vi "QCA INIT.vi"   [LabVIEW 2019]
doc: "INIT all sections of the QCA. This causes all config files to be reread and all configuration globals written to as if from power up."
uses:
  TPS Global.vi
  QCA Global.vi
  <vilib>/Utility/config.llb/Read Key (Path).vi
  <vilib>/Utility/config.llb/NI_LVConfig.lvlib
types:
  T1 = typedef "NI_LVConfig.lvlib/Config Data RefNum.ctl" = refnum<k1>
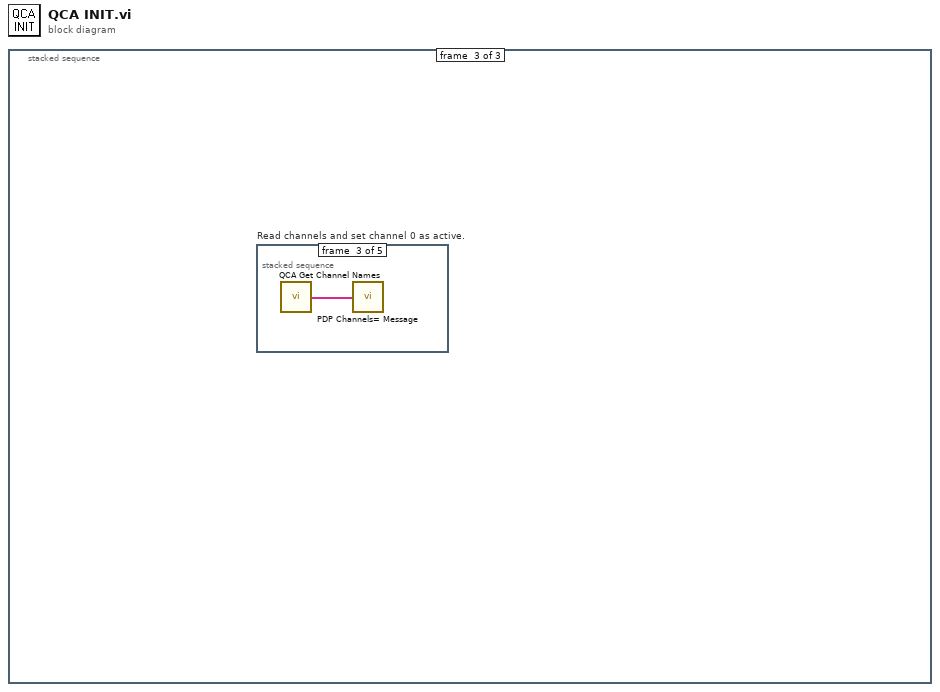
[diagram p0: block diagram]
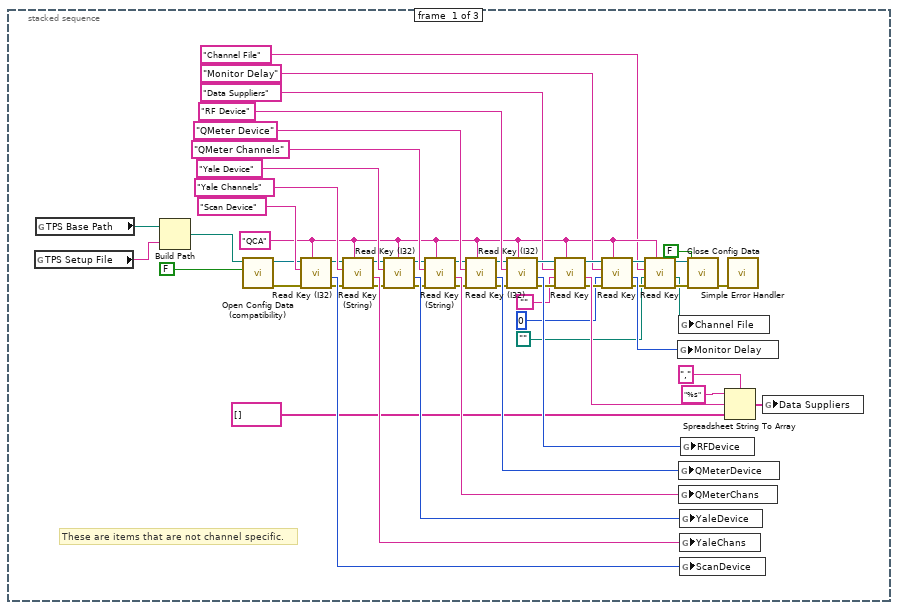
[diagram p2: hidden frame]
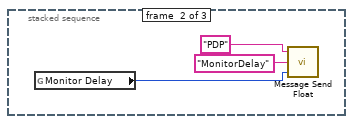
[diagram p3: hidden frame]
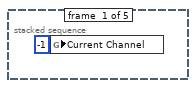
[diagram p4: hidden frame]
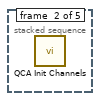
[diagram p5: hidden frame]
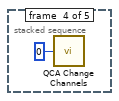
[diagram p6: hidden frame]
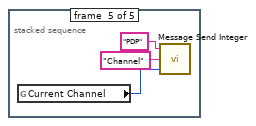
[diagram p7: hidden frame]
diagram:
  n1 = stacked-sequence {
    frame #0 {
      w5 = "QCA" ("section")
      # "These are items that are not channel specific."
      n2 = global read "TPS Global.vi" "TPS Setup File"() -> (w52:string)
      n3 = global read "TPS Global.vi" "TPS Base Path"() -> (w46:path)
      n4 = Build Path(base path=w46, name or relative path=w52) -> (appended path=w47:path)
      n5 = call <vilib>:"Open Config Data (compatibility).vi"("create file if necessary (T)"=FALSE ("create file if necessary? (T)"), "configuration file path"=w47) -> ("error out"=w49:errorcluster, "refnum"=w50:T1)  [unwired: 7 in, 1 out]
      n6 = call <vilib>:"Read Key (I32).vi"("section"=w5, "error in (no error)"=w49, "key"="Scan Device", "refnum"=w50) -> ("error out"=w34:errorcluster, "value"=w45:i32, "refnum out"=w24:T1)  [unwired: 4 in, 1 out]
      n7 = call <vilib>:"Read Key (String).vi"("section"=w5, "error in (no error)"=w34, "key"="Yale Channels", "refnum"=w24) -> ("error out"=w33:errorcluster, "value"=w44:string, "refnum out"=w25:T1)  [unwired: 4 in, 1 out]
      n8 = call <vilib>:"Read Key (I32).vi"("section"=w5, "error in (no error)"=w33, "key"="Yale Device", "refnum"=w25) -> ("error out"=w32:errorcluster, "value"=w41:i32, "refnum out"=w26:T1)  [unwired: 4 in, 1 out]
      n9 = call <vilib>:"Read Key (String).vi"("section"=w5, "error in (no error)"=w32, "key"="QMeter Channels", "refnum"=w26) -> ("error out"=w31:errorcluster, "value"=w40:string, "refnum out"=w27:T1)  [unwired: 4 in, 1 out]
      n10 = call <vilib>:"Read Key (I32).vi"("section"=w5, "error in (no error)"=w31, "key"="QMeter Device", "refnum"=w27) -> ("error out"=w30:errorcluster, "value"=w37:i32, "refnum out"=w28:T1)  [unwired: 4 in, 1 out]
      n11 = call <vilib>:"Read Key (I32).vi"("section"=w5, "error in (no error)"=w30, "key"="RF Device", "refnum"=w28) -> ("error out"=w23:errorcluster, "value"=w36:i32, "refnum out"=w22:T1)  [unwired: 4 in, 1 out]
      n12 = call-poly <vilib>:"Read Key.vi"("section"=w5, "error in (no error)"=w23, "default value"="", "key"="Data Suppliers", "refnum"=w22) -> ("error out"=w15:errorcluster, "value"=w19:string, "refnum out"=w14:T1)  [unwired: 3 in, 1 out]
      n13 = call-poly <vilib>:"Read Key.vi"("section"=w5, "error in (no error)"=w15, "default value"=0, "key"="Monitor Delay", "refnum"=w14) -> ("error out"=w9:errorcluster, "value"=w11:i32, "refnum out"=w8:T1)  [unwired: 3 in, 1 out]
      n14 = call-poly <vilib>:"Read Key.vi"("section"=w5, "error in (no error)"=w9, "default value"=path "", "key"="Channel File", "refnum"=w8) -> ("error out"=w7:errorcluster, "value"=w3:path, "refnum out"=w6:T1)  [unwired: 3 in, 1 out]
      n15 = global write "QCA Global.vi" "Monitor Delay"(w11) -> ()
      n16 = global write "QCA Global.vi" "Channel File"(w3) -> ()
      n17 = global write "QCA Global.vi" "QMeterDevice"(w37) -> ()
      n18 = global write "QCA Global.vi" "QMeterChans"(w40) -> ()
      n19 = global write "QCA Global.vi" "YaleDevice"(w41) -> ()
      n20 = global write "QCA Global.vi" "YaleChans"(w44) -> ()
      n21 = global write "QCA Global.vi" "ScanDevice"(w45) -> ()
      n22 = global write "QCA Global.vi" "RFDevice"(w36) -> ()
      n23 = call <vilib>:"Close Config Data.vi"("error in (no error)"=w7, "write file if changed (T)"=FALSE, "refnum"=w6) -> ("error out"=w29:errorcluster)  [unwired: 7 in, 1 out]
      n24 = Spreadsheet String To Array(delimiter (Tab)=",", format string="%s", spreadsheet string=w19, array type (2D Dbl)=string[] [] ("Array Constant")) -> (array=w16:string[])
      n25 = call <vilib>:"Simple Error Handler.vi"("error in (no error)"=w29) -> ()  [unwired: 4 in, 5 out]
      n26 = global write "QCA Global.vi" "Data Suppliers"(w16) -> ()
    }
    frame #1 {
      n27 = global read "QCA Global.vi" "Monitor Delay"() -> (w53:i32)
      n28 = call "Message Send Float.vi"("Value"=w53, "Parameter"="MonitorDelay", "Destination"="PDP") -> ()
    }
    frame #2 {
      n29 = stacked-sequence "Read channels and set channel 0 as active." {
        frame #0 {
          n30 = global write "QCA Global.vi" "Current Channel"(-1 ("Current Channel")) -> ()
        }
        frame #1 {
          n31 = call "QCA Init Channels.vi"() -> ()  [unwired: 1 in]
        }
        frame #2 {
          n32 = call "QCA Get Channel Names.vi"() -> ("Channel Names"=w57:string[])
          n33 = call "PDP Channels= Message.vi"("Channel"=w57) -> ()
        }
        frame #3 {
          n34 = call "QCA Change Channels.vi"("Channel"=0) -> ()
        }
        frame #4 {
          n35 = global read "QCA Global.vi" "Current Channel"() -> (w61:i32)
          n36 = call "Message Send Integer.vi"("Value"=w61, "Parameter"="Channel", "Destination"="PDP") -> ()
        }
      }
    }
  }
